vi "Initialize Virtual Camera.vi"(8 "error in (no error)":errorcluster, 11 "Application in":refnum<class "Application.lvclass">) -> (0 "error out":errorcluster, 3 "Application out":refnum<class "Application.lvclass">)   [LabVIEW 2018, in "Application.lvlib" / "Application.lvclass"]
uses:
  Application.lvclass
  C:/Program Files/National Instruments/LabVIEW 2018/vi.lib/ActorFramework/Actor/Actor.lvclass
  Hardware/Virtual Camera/Virtual Camera.lvclass
  Application.lvclass/Application.ctl
  <vilib>/ActorFramework/Actor/Actor.lvclass
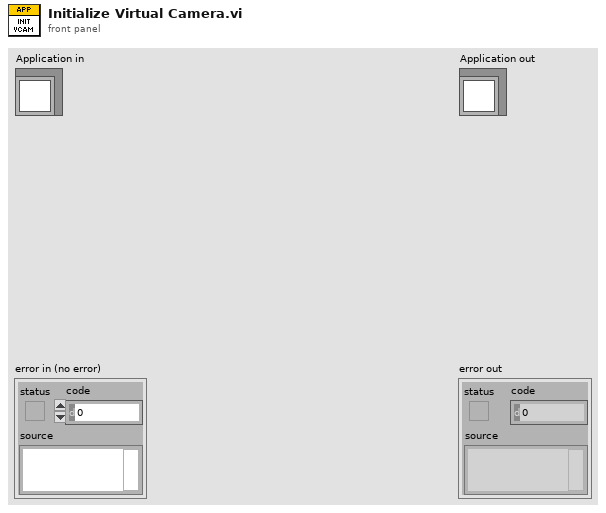
[diagram p1: front panel]
types:
  T1 = typedef "Virtual Camera Configuration.ctl" = cluster{"Camera Type":T2, "Active Cameras":T3[], "Sync Line":tag}
  T2 = typedef "Camera Type.ctl" = enum16{"Orca-Flash 4.0 V2"}
  T3 = typedef "Physical Camera Assignment.ctl" = cluster{"Channel Name":string, "Camera Type":T2, "Serial Number":string, "Flip Vertically":bool, "Flip Horizontally":bool, "photonsPerCount":dbl, "wavelength":i16}
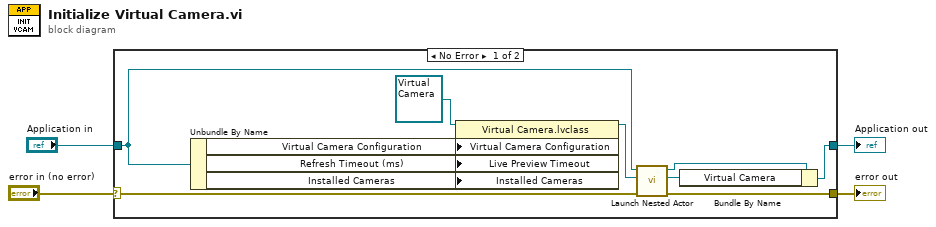
[diagram p0: block diagram]
diagram:
  n1 = case shown="No Error" "error in (no error)" {
    selector: "error in (no error)" -> [w5 w17]
    tunnel: [w13 w17] -> w3
    tunnel: [w14 w16] -> w1
    tunnel: "Application in" -> [w10 w16]
    frame No Error {
      n2 = Unbundle By Name(w10) -> ("Virtual Camera Configuration"=w7:T1, "Refresh Timeout (ms)"=w8:i32, "Installed Cameras"=w6:T3[])
      n3 = property class="Virtual Camera.lvclass"(reference=refnum<class "Virtual Camera.lvclass"> refnum ("Virtual Camera.lvlib:Virtual Camera.lvclass"), "Virtual Camera Configuration"=w7, "Live Preview Timeout"=w8, "Installed Cameras"=w6) -> (reference out=w11:refnum<class "Virtual Camera.lvclass">)  [unwired: 1 in, 1 out]
      n4 = call <vilib>:"Launch Nested Actor.vi"("error in (no error)"=w5, "Nested Actor"=w11, "Caller Actor in"=w10) -> ("error out"=w13:errorcluster, "Nested Actor's Enqueuer"=w15:refnum<class "Message Enqueuer.lvclass">, "Caller Actor out"=w9:refnum<class "Application.lvclass">)  [unwired: 6 in]
      n5 = Bundle By Name(cluster=w9, "Virtual Camera"=w15) -> (w14:refnum<class "Application.lvclass">)
    }
    frame Error {
    }
  }
  "error out" <- w3
  "Application out" <- w1
